vi "klastry.vi"(9 "reference 3":refnum<vi>, 10 "reference in":refnum<vi>, 11 "Cluster in":refnum<vi>) -> ()   [LabVIEW 2016]
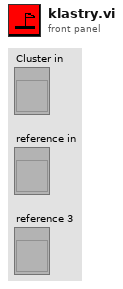
[diagram p1: front panel]
types:
  T1 = cluster{"Boolean 6":bool, "Boolean 6":bool, "Boolean 7":bool, "Boolean 8":bool, "Boolean 9":bool, "Boolean 10":bool, "Boolean 11":bool, "Boolean 12":bool, "Boolean 13":bool, "Boolean 14":bool, "Boolean 15":bool, "Boolean 16":bool, "Boolean 17":bool, "Boolean 18":bool, "Boolean 19":bool, "Boolean 20":bool, "Boolean 21":bool, "Boolean 22":bool, "Boolean 23":bool, "Boolean 24":bool, "Boolean 25":bool, "Boolean 26":bool, "Boolean 27":bool, "Boolean 28":bool, "Boolean 29":bool, "Boolean 30":bool, "Boolean 31":bool, "Boolean 32":bool, "Boolean 33":bool, "Boolean 34":bool, "Boolean 35":bool, "Boolean 36":bool, "Boolean 37":bool, "Boolean 38":bool, "Boolean 39":bool, "Boolean 40":bool, "Boolean 41":bool, "Boolean 42":bool, "Boolean 43":bool, "Boolean 44":bool, "Boolean 45":bool, "Boolean 46":bool, "Boolean 47":bool, "Boolean 48":bool, "Boolean 49":bool, "Boolean 50":bool, "Boolean 51":bool, "Boolean 52":bool, "Boolean 53":bool, "Boolean 54":bool, "Boolean 55":bool, "Boolean 56":bool, "Boolean 57":bool, "Boolean 58":bool, "Boolean 59":bool, "Boolean 60":bool, "Boolean 61":bool, "Boolean 62":bool, "Boolean 63":bool, "Boolean 64":bool, "Boolean 65":bool, "Boolean 66":bool, "Boolean 67":bool, "Boolean 68":bool, "Boolean 69":bool, "Boolean 70":bool, "Boolean 71":bool, "Boolean 72":bool, "Boolean 73":bool, "Boolean 74":bool, "Boolean 75":bool, "Boolean 76":bool, "Boolean 77":bool, "Boolean 78":bool, "Boolean 79":bool, "Boolean 80":bool, "Boolean 81":bool, "Boolean 82":bool, "Boolean 83":bool, "Boolean 84":bool, "Boolean 85":bool, "Boolean 86":bool, "Boolean 87":bool, "Boolean 88":bool, "Boolean 89":bool, "Boolean 90":bool, "Boolean 91":bool, "Boolean 92":bool, "Boolean 93":bool, "Boolean 94":bool, "Boolean 95":bool, "Boolean 96":bool, "Boolean 97":bool, "Boolean 98":bool, "Boolean 99":bool, "Boolean 100":bool, "Boolean 101":bool, "Boolean 102":bool, "Boolean 103":bool, "Boolean 104":bool, "Boolean 105":bool, "Boolean 106":bool, "Boolean 107":bool, "Boolean 108":bool, "Boolean 109":bool, "Boolean 110":bool, "Boolean 111":bool, "Boolean 112":bool, "Boolean 113":bool, "Boolean 114":bool, "Boolean 115":bool, "Boolean 116":bool, "Boolean 117":bool, "Boolean 118":bool, "Boolean 119":bool, "Boolean 120":bool, "Boolean 121":bool, "Boolean 122":bool, "Boolean 123":bool, "Boolean 124":bool, "Boolean 125":bool, "Boolean 126":bool, "Boolean 127":bool, "Boolean 128":bool, "Boolean 129":bool, "Boolean 130":bool, "Boolean 131":bool, "Boolean 132":bool, "Boolean 133":bool, "Boolean 134":bool, "Boolean 135":bool, "Boolean 136":bool, "Boolean 137":bool, "Boolean 138":bool, "Boolean 139":bool, "Boolean 140":bool, "Boolean 141":bool, "Boolean 142":bool, "Boolean 143":bool, "Boolean 144":bool, "Boolean 145":bool, "Boolean 146":bool, "Boolean 147":bool, "Boolean 148":bool}
  T2 = cluster{"Boolean 6":bool, "Boolean 6":bool, "Boolean 7":bool, "Boolean 8":bool, "Boolean 9":bool, "Boolean 10":bool, "Boolean 11":bool, "Boolean 12":bool, "Boolean 17":bool, "Boolean 18":bool, "Boolean 19":bool, "Boolean 20":bool, "Boolean 21":bool, "Boolean 22":bool, "Boolean 23":bool, "Boolean 24":bool, "Boolean 29":bool, "Boolean 30":bool, "Boolean 31":bool, "Boolean 32":bool, "Boolean 33":bool, "Boolean 34":bool, "Boolean 35":bool, "Boolean 36":bool, "Boolean 41":bool, "Boolean 42":bool, "Boolean 43":bool, "Boolean 44":bool, "Boolean 45":bool, "Boolean 46":bool, "Boolean 47":bool, "Boolean 48":bool, "Boolean 53":bool, "Boolean 54":bool, "Boolean 55":bool, "Boolean 56":bool, "Boolean 57":bool, "Boolean 58":bool, "Boolean 59":bool, "Boolean 60":bool, "Boolean 65":bool, "Boolean 66":bool, "Boolean 67":bool, "Boolean 68":bool, "Boolean 69":bool, "Boolean 70":bool, "Boolean 71":bool, "Boolean 72":bool, "Boolean 77":bool, "Boolean 78":bool, "Boolean 79":bool, "Boolean 80":bool, "Boolean 81":bool, "Boolean 82":bool, "Boolean 83":bool, "Boolean 84":bool, "Boolean 89":bool, "Boolean 90":bool, "Boolean 91":bool, "Boolean 92":bool, "Boolean 93":bool, "Boolean 94":bool, "Boolean 95":bool, "Boolean 96":bool}
  T3 = cluster{"Boolean 6":bool, "Boolean 6":bool, "Boolean 7":bool, "Boolean 8":bool, "Boolean 9":bool, "Boolean 10":bool, "Boolean 17":bool, "Boolean 18":bool, "Boolean 19":bool, "Boolean 20":bool, "Boolean 21":bool, "Boolean 22":bool, "Boolean 29":bool, "Boolean 30":bool, "Boolean 31":bool, "Boolean 32":bool, "Boolean 33":bool, "Boolean 34":bool, "Boolean 41":bool, "Boolean 42":bool, "Boolean 43":bool, "Boolean 44":bool, "Boolean 45":bool, "Boolean 46":bool, "Boolean 53":bool, "Boolean 54":bool, "Boolean 55":bool, "Boolean 56":bool, "Boolean 57":bool, "Boolean 58":bool, "Boolean 65":bool, "Boolean 66":bool, "Boolean 67":bool, "Boolean 68":bool, "Boolean 69":bool, "Boolean 70":bool}
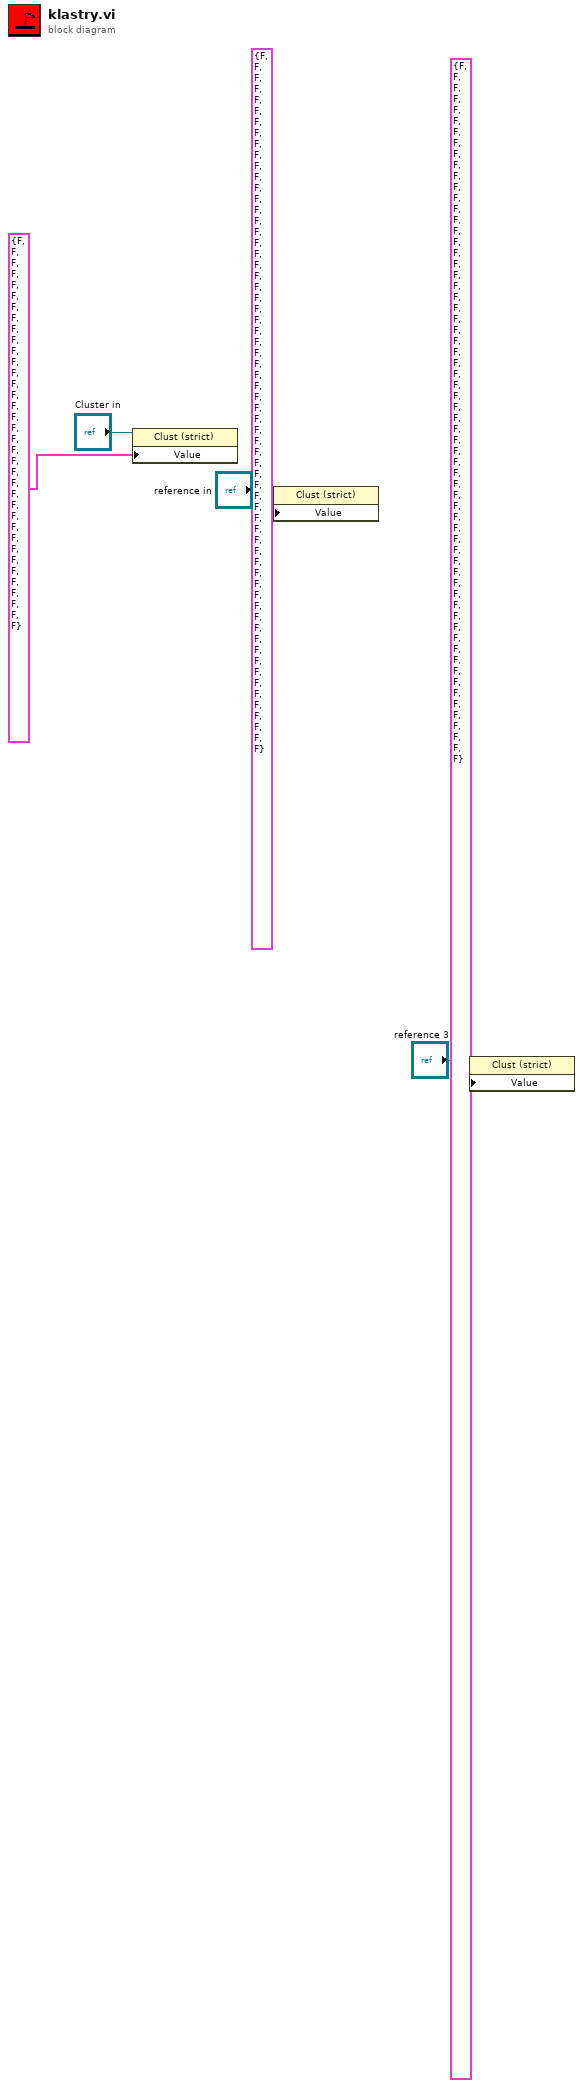
[diagram p0: block diagram]
diagram:
  n1 = property class="Clust (strict)"(reference="Cluster in", "Value"=T3 {"Boolean 6"=FALSE, "Boolean 6"=FALSE, "Boolean 7"=FALSE, "Boolean 8"=FALSE, "Boolean 9"=FALSE, "Boolean 10"=FALSE, "Boolean 17"=FALSE, "Boolean 18"=FALSE, "Boolean 19"=FALSE, "Boolean 20"=FALSE, "Boolean 21"=FALSE, "Boolean 22"=FALSE, "Boolean 29"=FALSE, "Boolean 30"=FALSE, "Boolean 31"=FALSE, "Boolean 32"=FALSE, "Boolean 33"=FALSE, "Boolean 34"=FALSE, "Boolean 41"=FALSE, "Boolean 42"=FALSE, "Boolean 43"=FALSE, "Boolean 44"=FALSE, "Boolean 45"=FALSE, "Boolean 46"=FALSE, "Boolean 53"=FALSE, "Boolean 54"=FALSE, "Boolean 55"=FALSE, "Boolean 56"=FALSE, "Boolean 57"=FALSE, "Boolean 58"=FALSE, "Boolean 65"=FALSE, "Boolean 66"=FALSE, "Boolean 67"=FALSE, "Boolean 68"=FALSE, "Boolean 69"=FALSE, "Boolean 70"=FALSE} ("Cluster 1")) -> ()  [unwired: 1 in, 2 out]
  n2 = property class="Clust (strict)"(reference="reference in", "Value"=T2 {"Boolean 6"=FALSE, "Boolean 6"=FALSE, "Boolean 7"=FALSE, "Boolean 8"=FALSE, "Boolean 9"=FALSE, "Boolean 10"=FALSE, "Boolean 11"=FALSE, "Boolean 12"=FALSE, "Boolean 17"=FALSE, "Boolean 18"=FALSE, "Boolean 19"=FALSE, "Boolean 20"=FALSE, "Boolean 21"=FALSE, "Boolean 22"=FALSE, "Boolean 23"=FALSE, "Boolean 24"=FALSE, "Boolean 29"=FALSE, "Boolean 30"=FALSE, "Boolean 31"=FALSE, "Boolean 32"=FALSE, "Boolean 33"=FALSE, "Boolean 34"=FALSE, "Boolean 35"=FALSE, "Boolean 36"=FALSE, "Boolean 41"=FALSE, "Boolean 42"=FALSE, "Boolean 43"=FALSE, "Boolean 44"=FALSE, "Boolean 45"=FALSE, "Boolean 46"=FALSE, "Boolean 47"=FALSE, "Boolean 48"=FALSE, "Boolean 53"=FALSE, "Boolean 54"=FALSE, "Boolean 55"=FALSE, "Boolean 56"=FALSE, "Boolean 57"=FALSE, "Boolean 58"=FALSE, "Boolean 59"=FALSE, "Boolean 60"=FALSE, "Boolean 65"=FALSE, "Boolean 66"=FALSE, "Boolean 67"=FALSE, "Boolean 68"=FALSE, "Boolean 69"=FALSE, "Boolean 70"=FALSE, "Boolean 71"=FALSE, "Boolean 72"=FALSE, "Boolean 77"=FALSE, "Boolean 78"=FALSE, "Boolean 79"=FALSE, "Boolean 80"=FALSE, "Boolean 81"=FALSE, "Boolean 82"=FALSE, "Boolean 83"=FALSE, "Boolean 84"=FALSE, "Boolean 89"=FALSE, "Boolean 90"=FALSE, "Boolean 91"=FALSE, "Boolean 92"=FALSE, "Boolean 93"=FALSE, "Boolean 94"=FALSE, "Boolean 95"=FALSE, "Boolean 96"=FALSE} ("Cluster 3")) -> ()  [unwired: 1 in, 2 out]
  n3 = property class="Clust (strict)"(reference="reference 3", "Value"=T1 {"Boolean 6"=FALSE, "Boolean 6"=FALSE, "Boolean 7"=FALSE, "Boolean 8"=FALSE, "Boolean 9"=FALSE, "Boolean 10"=FALSE, "Boolean 11"=FALSE, "Boolean 12"=FALSE, "Boolean 13"=FALSE, "Boolean 14"=FALSE, "Boolean 15"=FALSE, "Boolean 16"=FALSE, "Boolean 17"=FALSE, "Boolean 18"=FALSE, "Boolean 19"=FALSE, "Boolean 20"=FALSE, "Boolean 21"=FALSE, "Boolean 22"=FALSE, "Boolean 23"=FALSE, "Boolean 24"=FALSE, "Boolean 25"=FALSE, "Boolean 26"=FALSE, "Boolean 27"=FALSE, "Boolean 28"=FALSE, "Boolean 29"=FALSE, "Boolean 30"=FALSE, "Boolean 31"=FALSE, "Boolean 32"=FALSE, "Boolean 33"=FALSE, "Boolean 34"=FALSE, "Boolean 35"=FALSE, "Boolean 36"=FALSE, "Boolean 37"=FALSE, "Boolean 38"=FALSE, "Boolean 39"=FALSE, "Boolean 40"=FALSE, "Boolean 41"=FALSE, "Boolean 42"=FALSE, "Boolean 43"=FALSE, "Boolean 44"=FALSE, "Boolean 45"=FALSE, "Boolean 46"=FALSE, "Boolean 47"=FALSE, "Boolean 48"=FALSE, "Boolean 49"=FALSE, "Boolean 50"=FALSE, "Boolean 51"=FALSE, "Boolean 52"=FALSE, "Boolean 53"=FALSE, "Boolean 54"=FALSE, "Boolean 55"=FALSE, "Boolean 56"=FALSE, "Boolean 57"=FALSE, "Boolean 58"=FALSE, "Boolean 59"=FALSE, "Boolean 60"=FALSE, "Boolean 61"=FALSE, "Boolean 62"=FALSE, "Boolean 63"=FALSE, "Boolean 64"=FALSE, "Boolean 65"=FALSE, "Boolean 66"=FALSE, "Boolean 67"=FALSE, "Boolean 68"=FALSE, "Boolean 69"=FALSE, "Boolean 70"=FALSE, "Boolean 71"=FALSE, "Boolean 72"=FALSE, "Boolean 73"=FALSE, "Boolean 74"=FALSE, "Boolean 75"=FALSE, "Boolean 76"=FALSE, "Boolean 77"=FALSE, "Boolean 78"=FALSE, "Boolean 79"=FALSE, "Boolean 80"=FALSE, "Boolean 81"=FALSE, "Boolean 82"=FALSE, "Boolean 83"=FALSE, "Boolean 84"=FALSE, "Boolean 85"=FALSE, "Boolean 86"=FALSE, "Boolean 87"=FALSE, "Boolean 88"=FALSE, "Boolean 89"=FALSE, "Boolean 90"=FALSE, "Boolean 91"=FALSE, "Boolean 92"=FALSE, "Boolean 93"=FALSE, "Boolean 94"=FALSE, "Boolean 95"=FALSE, "Boolean 96"=FALSE, "Boolean 97"=FALSE, "Boolean 98"=FALSE, "Boolean 99"=FALSE, "Boolean 100"=FALSE, "Boolean 101"=FALSE, "Boolean 102"=FALSE, "Boolean 103"=FALSE, "Boolean 104"=FALSE, "Boolean 105"=FALSE, "Boolean 106"=FALSE, "Boolean 107"=FALSE, "Boolean 108"=FALSE, "Boolean 109"=FALSE, "Boolean 110"=FALSE, "Boolean 111"=FALSE, "Boolean 112"=FALSE, "Boolean 113"=FALSE, "Boolean 114"=FALSE, "Boolean 115"=FALSE, "Boolean 116"=FALSE, "Boolean 117"=FALSE, "Boolean 118"=FALSE, "Boolean 119"=FALSE, "Boolean 120"=FALSE, "Boolean 121"=FALSE, "Boolean 122"=FALSE, "Boolean 123"=FALSE, "Boolean 124"=FALSE, "Boolean 125"=FALSE, "Boolean 126"=FALSE, "Boolean 127"=FALSE, "Boolean 128"=FALSE, "Boolean 129"=FALSE, "Boolean 130"=FALSE, "Boolean 131"=FALSE, "Boolean 132"=FALSE, "Boolean 133"=FALSE, "Boolean 134"=FALSE, "Boolean 135"=FALSE, "Boolean 136"=FALSE, "Boolean 137"=FALSE, "Boolean 138"=FALSE, "Boolean 139"=FALSE, "Boolean 140"=FALSE, "Boolean 141"=FALSE, "Boolean 142"=FALSE, "Boolean 143"=FALSE, "Boolean 144"=FALSE, "Boolean 145"=FALSE, "Boolean 146"=FALSE, "Boolean 147"=FALSE, "Boolean 148"=FALSE} ("Cluster 4")) -> ()  [unwired: 1 in, 2 out]
